vi "reset.vi"(8 "error in (no error)":errorcluster, 11 "SignalReaderDL091205FPGA in":refnum<class "SignalReaderDL091205FPGA.lvclass">) -> (0 "error out":errorcluster, 3 "SignalReaderDL091205FPGA out":refnum<class "SignalReaderDL091205FPGA.lvclass">)   [LabVIEW 2010, in "SignalReaderDL091205FPGA.lvclass"]
uses:
  SignalReaderDL091205FPGA.lvclass
  SignalReaderDL091205FPGA.lvclass/SignalReaderDL091205FPGA.ctl
  FPGAWrapper/GenericFPGAWrapper/GenericFPGAWrapper/GenericFPGAWrapper.lvclass
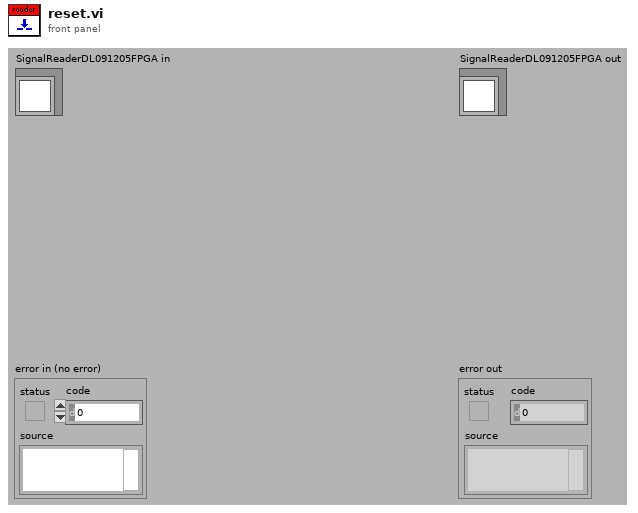
[diagram p1: front panel]
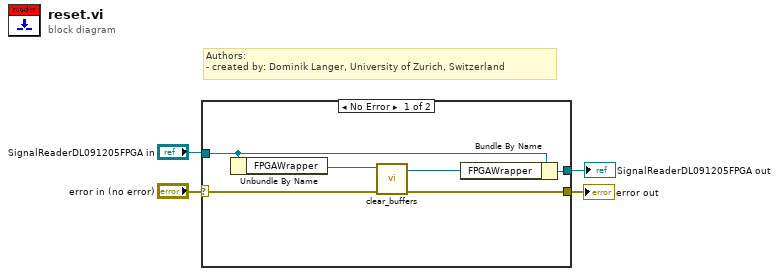
[diagram p0: block diagram]
diagram:
  # "Authors: \n- created by: Dominik Langer, University of Zurich, Switzerland"
  n1 = case shown="No Error" "error in (no error)" {
    selector: "error in (no error)" -> [w8 w12]
    tunnel: [w6 w12] -> w2
    tunnel: [w9 w11] -> w1
    tunnel: "SignalReaderDL091205FPGA in" -> [w10 w11]
    frame No Error {
      n2 = Unbundle By Name(w10) -> ("FPGAWrapper"=w7:refnum<class "GenericFPGAWrapper.lvclass">)
      n3 = call-dynamic "clear_buffers.vi"("error in (no error)"=w8, "GenericFPGAWrapper in"=w7) -> ("error out"=w6:errorcluster, "GenericFPGAWrapper out"=w5:refnum<class "GenericFPGAWrapper.lvclass">)  [unwired: 8 out]
      n4 = Bundle By Name(cluster=w10, "FPGAWrapper"=w5) -> (w9:refnum<class "SignalReaderDL091205FPGA.lvclass">)
    }
    frame Error {
    }
  }
  "error out" <- w2
  "SignalReaderDL091205FPGA out" <- w1
